vi "UDPTester.vi"() -> ()   [LabVIEW 2013]
uses:
  <vilib>/Utility/tcp.llb/UDP Multicast Write-Only Open.vi
panel:
  in  "Stop Button":bool
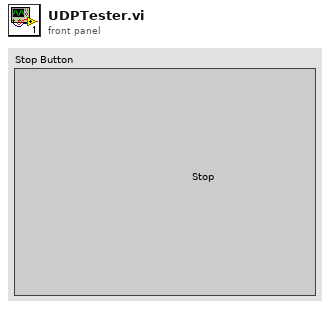
[diagram p1: front panel]
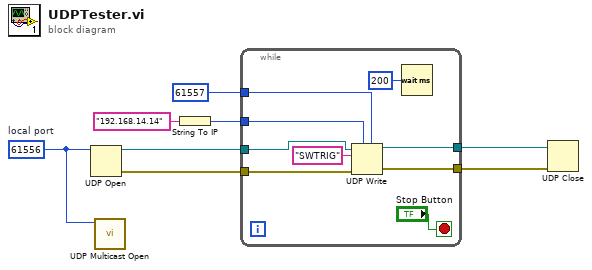
[diagram p0: block diagram]
diagram:
  w1 = u16 61556  # local port
  n1 = UDP Open(11:w1) -> (port=w5:refnum<k16>, 0:w4:errorcluster)  [unwired: 4 in, 1 out]
  n2 = call-poly <vilib>:"UDP Multicast Open.vi"("port"=w1) -> ()  [unwired: 9 in, 2 out]
  n3 = String To IP(1:"192.168.14.14" ("name")) -> (0:w7:u32)
  n4 = while {
    tunnel: w7 -> [w17]
    tunnel: u16 61557 ("port") -> [w16]
    tunnel: w5 -> [w14]
    tunnel: w4 -> [w13]
    tunnel: [w11] -> w3
    tunnel: [w10] -> w2
    stop <- "Stop Button" stop-if-true
    n5 = UDP Write(address=w17, port or service name=w16, connection ID=w14, data in="SWTRIG", 8:w13) -> (error out=w11:errorcluster, 3:w10:refnum<k16>)  [unwired: 1 in]
    n6 = Wait (ms)(milliseconds to wait=u32 200) -> ()  [unwired: 1 out]
  }
  n7 = UDP Close(connection ID=w2, 8:w3) -> ()  [unwired: 2 out]
